vi "GetFilesPCI.vi"(4 "error in (no error)":errorcluster, 6 "Test Num :":u32, 7 "Project :":string) -> (0 "error out":errorcluster, 3 "NomProjetOut":string)   [LabVIEW 2017]
uses:
  DefDeType/WhichPath.ctl
panel:
  out "Glissière":i32(slide) scale=0.0..100.0
  out "noms des fichiers":string[](array[string])
  out "HBM File":bool
  out "Qualisys file":bool
  out "PCI file":bool
  in  "Etat":string
  # "Files Check"
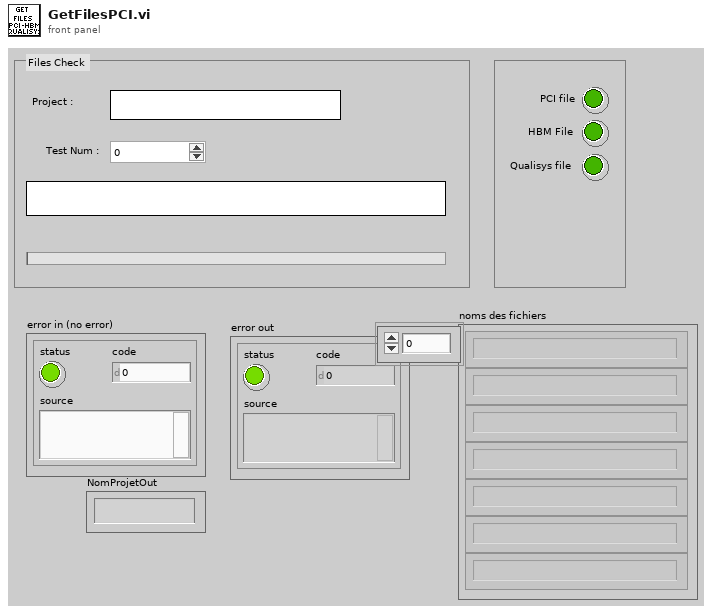
[diagram p1: front panel]
types:
  T1 = typedef "WhichPath.ctl" = enum16{"DossierProjet", "Config", "Meas", "MeasPCI", "MeasCRIO1", "MeasCRIO2", "MeasQualisys", "MeasHBM", "MeasTDMS", "Fig", "Res"}
  T2 = typedef "ConfigTotale.ctl" = cluster{"VoltageChannels":T3, "WheastoneBridgeChannels":T4, "Configuration":T5}
  T3 = typedef "VoltageChannels.ctl" = cluster{"ChannelNames":string[], "Sensitivity(Unit/V)":dbl[], "AutoZero":bool[], "ChannelUnits":string[], "Offsets(Units)":dbl[], "Graph Num":u8[]}
  T4 = typedef "WBridgeChannels.ctl" = cluster{"ChannelNames":string[], "Sensitivity(Unit/V)":dbl[], "AutoZero":bool[], "ChannelUnits":string[], "Offsets(Units)":dbl[], "Graph Num":u8[]}
  T5 = typedef "Configuration.ctl" = cluster{"AcqSamplingRate(Hz)":u32, "AcqTime(s)":u32, "Trigger":bool, "NbVoltageChannels":u32, "NbWBridgeChannels":u32, "Qualisys":bool, "Hexapode":bool, "FinalSamplingRate(Hz)":u32, "QualisysDataType":enum16{"6DOF", "3DTracking", "6DOF + 3D"}, "Nortek":bool, "HBM":bool}
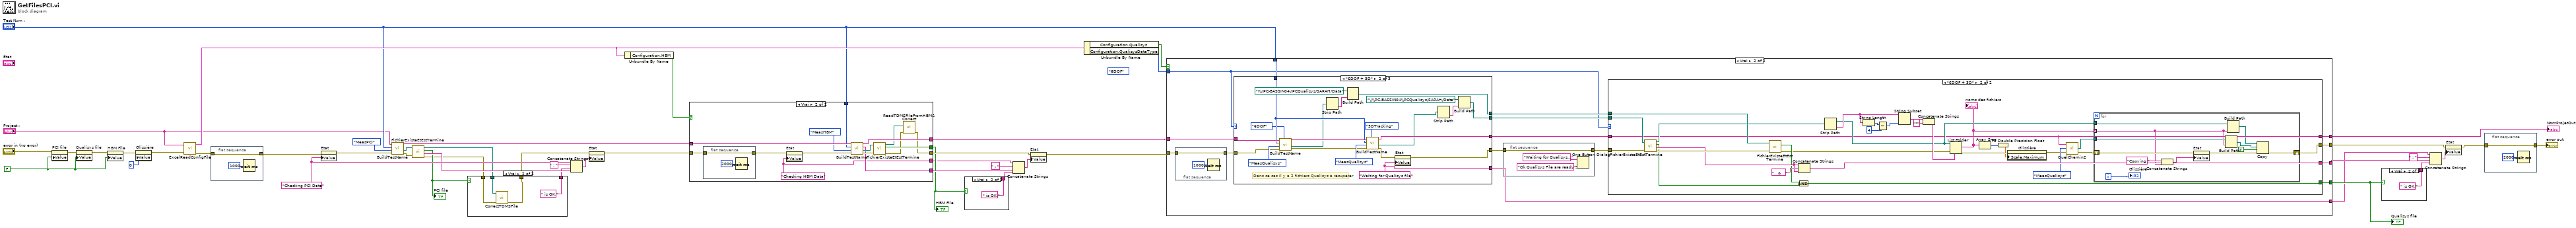
[diagram p0: block diagram]
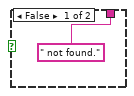
[diagram p2: hidden frame]
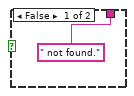
[diagram p3: hidden frame]
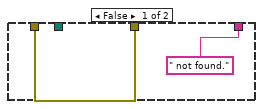
[diagram p4: hidden frame]
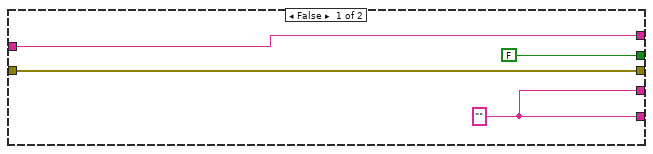
[diagram p5: hidden frame]
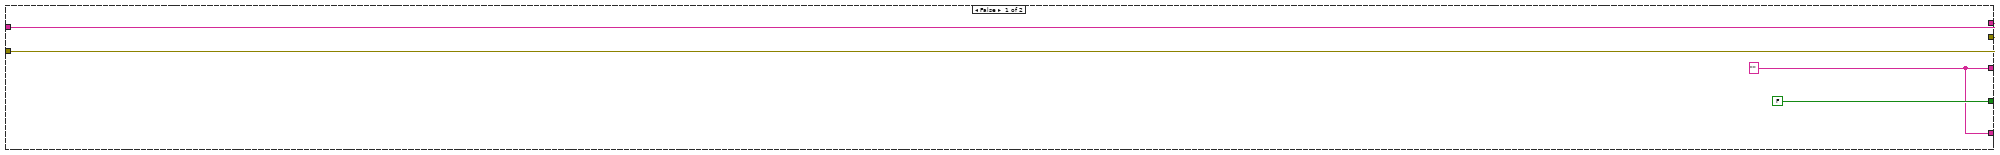
[diagram p6: hidden frame]
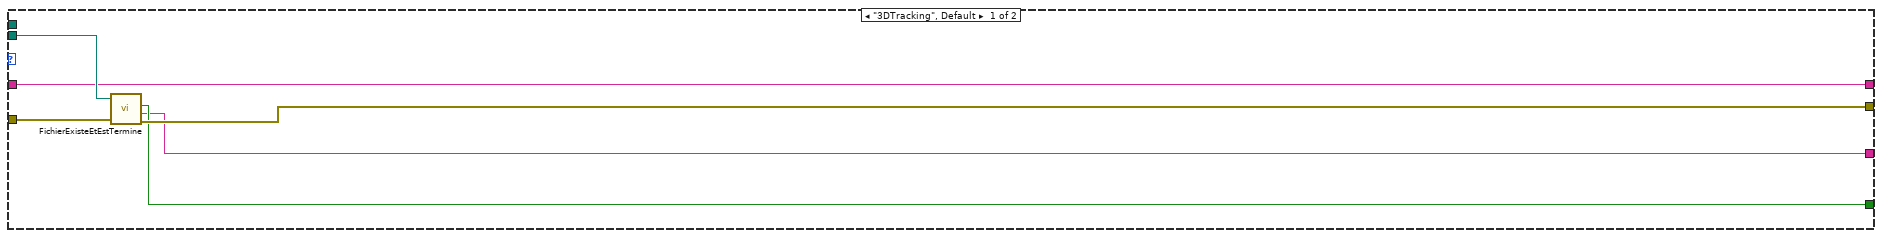
[diagram p7: hidden frame]
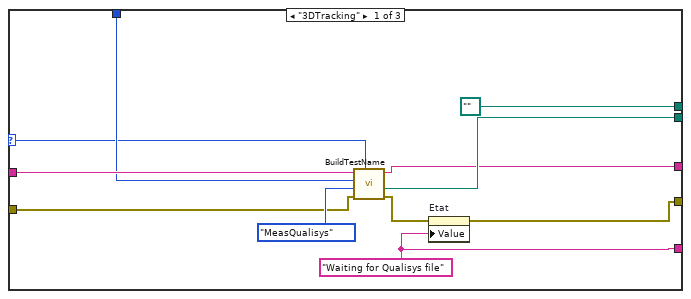
[diagram p8: hidden frame]
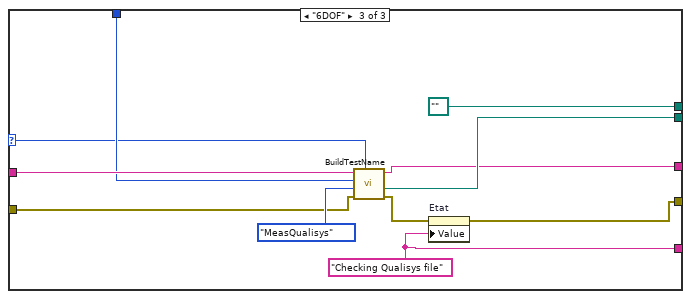
[diagram p9: hidden frame]
diagram:
  w27 = "Checking PCI Data" ("Etat")
  (unwired) enum16{"6DOF", "3DTracking", "6DOF + 3D"}."6DOF" ("Configuration.QualisysDataType")
  w38 = FALSE ("Valise file")
  n1 = property on="PCI file" class="Bool (strict)"(error in="error in (no error)", "Value"=w38) -> (error out=w48:errorcluster)  [unwired: 1 in, 1 out]
  n2 = property on="Qualisys file" class="Bool (strict)"(error in=w48, "Value"=w38) -> (error out=w39:errorcluster)  [unwired: 1 in, 1 out]
  n3 = property on="HBM File" class="Bool (strict)"(error in=w39, "Value"=w38) -> (error out=w3:errorcluster)  [unwired: 1 in, 1 out]
  n4 = property on="Glissière" class="Gliss (strict)"(error in=w3, "Value"=0 ("Glissière")) -> (error out=w2:errorcluster)  [unwired: 1 in, 1 out]
  n5 = call "ExcelReadConfigFile.vi"("NomProjet"="Project :", "error in (no error)"=w2) -> ("ConfigurationTotale"=w41:T2, "error out"=w44:errorcluster)  [unwired: 3 in]
  n6 = flat-sequence {
    tunnel: w44 -> [w51]
    tunnel: [w51] -> w31
    frame #0 {
      n7 = Wait (ms)(milliseconds to wait=u32 1000) -> ()  [unwired: 1 out]
    }
  }
  n8 = property on="Etat" class="Ch"(error in=w31, "Value"=w27) -> (error out=w30:errorcluster)  [unwired: 1 in, 1 out]
  n9 = call "BuildTestName.vi"("entrée d'erreur"=w30, "WhichPath?"=WhichPath."MeasPCI", "NextTestNum"="Test Num :", "NomProjet"="Project :") -> ("sortie d'erreur"=w33:errorcluster, "cheminProchainFichier"=w32:path, "NomProjetOut"=w34:string)  [unwired: 1 in, 1 out]
  n10 = call "FichierExisteEtEstTermine.vi"("cheminProchainFichierRAW"=w32, "entrée d'erreur (pas d'erreur)"=w33) -> ("path out"=w6:path, "ExisteEtTermine"=w23:bool, "nomFichier"=w25:string, "sortie d'erreur"=w5:errorcluster)  [unwired: 1 in]
  "PCI file" <- w23
  n11 = case shown="Vrai" w23 {
    tunnel: [" not found." ("chaîne") " is OK." ("chaîne")] -> w24
    tunnel: w6 -> [_ w54]
    tunnel: w5 -> [w52 w56]
    tunnel: [w52 w55] -> w4
    frame False {
    }
    frame True {
      n12 = call "CorrectTDMSFile.vi"("entrée d'erreur (pas d'erreur)"=w56, "chemin du fichier"=w54) -> ("sortie d'erreur"=w55:errorcluster)  [unwired: 5 in]
    }
  }
  n13 = Concatenate Strings(w27, " : " ("chaîne"), w25, w24) -> (w28:string)
  n14 = property on="Etat" class="Ch"(error in=w4, "Value"=w28) -> (error out=w29:errorcluster)  [unwired: 1 in, 1 out]
  n15 = Unbundle By Name(w41) -> ("Configuration.HBM"=w43:bool)
  n16 = case shown="Vrai" w43 {
    tunnel: w29 -> [w61 w72]
    tunnel: [w61 w63] -> w19
    tunnel: [w60 w70] -> w40
    tunnel: w34 -> [w60 w76]
    tunnel: "Test Num :" -> [_ w74]
    tunnel: [FALSE ("ExisteEtTermine") w67] -> w16
    tunnel: [w58 w66] -> w17
    tunnel: [w58 w65] -> w8
    frame False {
      w58 = "" ("NomProchainFichier")
    }
    frame True {
      w65 = "Checking HBM Data" ("Etat")
      n17 = flat-sequence {
        tunnel: w72 -> [w78]
        tunnel: [w78] -> w73
        frame #0 {
          n18 = Wait (ms)(milliseconds to wait=u32 2000) -> ()  [unwired: 1 out]
        }
      }
      n19 = property on="Etat" class="Ch"(error in=w73, "Value"=w65) -> (error out=w75:errorcluster)  [unwired: 1 in, 1 out]
      n20 = call "BuildTestName.vi"("entrée d'erreur"=w75, "WhichPath?"=WhichPath."MeasHBM", "NextTestNum"=w74, "NomProjet"=w76) -> ("sortie d'erreur"=w68:errorcluster, "cheminProchainFichier"=w69:path, "NomProchainFichier"=w66:string, "NomProjetOut"=w70:string)  [unwired: 1 in]
      n21 = call "FichierExisteEtEstTermine.vi"("cheminProchainFichierRAW"=w69, "entrée d'erreur (pas d'erreur)"=w68) -> ("path out"=w62:path, "ExisteEtTermine"=w67:bool, "sortie d'erreur"=w64:errorcluster)  [unwired: 1 in, 1 out]
      n22 = call "ReadTDMSFileFromHBM&Correct.vi"("error in (no error)"=w64, "file path"=w62) -> ("sortie d'erreur"=w63:errorcluster)  [unwired: 4 in, 1 out]
    }
  }
  "HBM File" <- w16
  n23 = case shown="Vrai" w16 {
    tunnel: [" not found." ("chaîne") " is OK." ("chaîne")] -> w22
    frame False {
    }
    frame True {
    }
  }
  n24 = Concatenate Strings(w8, " : " ("chaîne"), w17, w22) -> (w20:string)
  n25 = property on="Etat" class="Ch"(error in=w19, "Value"=w20) -> (error out=w18:errorcluster)  [unwired: 1 in, 1 out]
  n26 = Unbundle By Name(w41) -> ("Configuration.Qualisys"=w47:bool, "Configuration.QualisysDataType"=w45:enum16{"6DOF", "3DTracking", "6DOF + 3D"})
  n27 = case shown="Vrai" w47 {
    tunnel: w18 -> [w84 w93]
    tunnel: w40 -> [w83 w97]
    tunnel: w45 -> [_ w90]
    tunnel: "Test Num :" -> [_ w96]
    tunnel: [w84 w95] -> w12
    tunnel: [w83 w94] -> w42
    tunnel: [w81 w87] -> w10
    tunnel: [FALSE ("ExisteEtTermine") w89] -> w9
    tunnel: [w81 w88] -> w7
    frame False {
      w81 = "" ("nomFichier")
    }
    frame True {
      n28 = flat-sequence {
        tunnel: w93 -> [w195]
        tunnel: [w195] -> w92
        frame #0 {
          n29 = Wait (ms)(milliseconds to wait=u32 1000) -> ()  [unwired: 1 out]
        }
      }
      n30 = case shown="\"6DOF + 3D\"" w90 {
        selector: w90 -> [w153 _ w185]
        tunnel: [w161 w162 w193] -> w99
        tunnel: [w160 w182 w192] -> w86
        tunnel: [w159 w181 w191] -> w98
        tunnel: w97 -> [w156 w174 w188]
        tunnel: w96 -> [w155 w173 w187]
        tunnel: w92 -> [w154 w176 w186]
        tunnel: [path "" ("cheminProchainFichier") w166 path "" ("cheminProchainFichier")] -> w91
        tunnel: [w151 w170 w183] -> w88
        frame "3DTracking" {
          w151 = "Waiting for Qualisys file" ("Etat")
          n31 = call "BuildTestName.vi"("QualisysDataType"=w153, "entrée d'erreur"=w154, "WhichPath?"=WhichPath."MeasQualisys", "NextTestNum"=w155, "NomProjet"=w156) -> ("sortie d'erreur"=w157:errorcluster, "cheminProchainFichier"=w161:path, "NomProjetOut"=w159:string)  [unwired: 1 out]
          n32 = property on="Etat" class="Ch"(error in=w157, "Value"=w151) -> (error out=w160:errorcluster)  [unwired: 1 in, 1 out]
        }
        frame "6DOF + 3D" {
          w170 = "Waiting for Qualisys file" ("Etat")
          # "Dans ce cas il y a 2 fichiers Qualisys à récupérer"
          n33 = call "BuildTestName.vi"("QualisysDataType"=enum16{"6DOF", "3DTracking", "6DOF + 3D"}."6DOF", "entrée d'erreur"=w176, "WhichPath?"=WhichPath."MeasQualisys", "NextTestNum"=w173, "NomProjet"=w174) -> ("sortie d'erreur"=w177:errorcluster, "cheminProchainFichier"=w168:path, "NomProjetOut"=w175:string)  [unwired: 1 out]
          n34 = Strip Path(path=w168) -> (name=w167:string)  [unwired: 1 out]
          n35 = Build Path(base path=path "\\\\PC-BASSIN04\\PCQualisys/SARAH/Data" ("chemin de base"), name or relative path=w167) -> (appended path=w166:path)
          n36 = call "BuildTestName.vi"("QualisysDataType"=enum16{"6DOF", "3DTracking", "6DOF + 3D"}."3DTracking", "entrée d'erreur"=w177, "WhichPath?"=WhichPath."MeasQualisys", "NextTestNum"=w173, "NomProjet"=w175) -> ("sortie d'erreur"=w179:errorcluster, "cheminProchainFichier"=w163:path, "NomProjetOut"=w181:string)  [unwired: 1 out]
          n37 = property on="Etat" class="Ch"(error in=w179, "Value"=w170) -> (error out=w182:errorcluster)  [unwired: 1 in, 1 out]
          n38 = Strip Path(path=w163) -> (name=w165:string)  [unwired: 1 out]
          n39 = Build Path(base path=path "\\\\PC-BASSIN04\\PCQualisys/SARAH/Data" ("chemin de base"), name or relative path=w165) -> (appended path=w162:path)
        }
        frame "6DOF" {
          w183 = "Checking Qualisys file" ("Etat")
          n40 = call "BuildTestName.vi"("QualisysDataType"=w185, "entrée d'erreur"=w186, "WhichPath?"=WhichPath."MeasQualisys", "NextTestNum"=w187, "NomProjet"=w188) -> ("sortie d'erreur"=w189:errorcluster, "cheminProchainFichier"=w193:path, "NomProjetOut"=w191:string)  [unwired: 1 out]
          n41 = property on="Etat" class="Ch"(error in=w189, "Value"=w183) -> (error out=w192:errorcluster)  [unwired: 1 in, 1 out]
        }
      }
      n42 = flat-sequence {
        tunnel: w86 -> [w102]
        tunnel: [w102] -> w85
        frame #0 {
          n43 = One Button Dialog(message="Waiting for Qualisys...", button name ("OK")="Ok Qualisys File are ready!!" ("nom du bouton (\"OK\")")) -> ()  [unwired: 1 out]
        }
      }
      n44 = case shown="\"6DOF + 3D\"" w90 {
        tunnel: w99 -> [w107 w136]
        tunnel: w85 -> [w108 w138]
        tunnel: w98 -> [w105 w117]
        tunnel: [w106 w120] -> w95
        tunnel: [w105 w117] -> w94
        tunnel: w91 -> [_ w135]
        tunnel: [w104 w129] -> w89
        tunnel: [w103 w132] -> w87
        frame "3DTracking", Default {
          n45 = call "FichierExisteEtEstTermine.vi"("cheminProchainFichierRAW"=w107, "entrée d'erreur (pas d'erreur)"=w108) -> ("ExisteEtTermine"=w104:bool, "nomFichier"=w103:string, "sortie d'erreur"=w106:errorcluster)  [unwired: 1 in, 1 out]
        }
        frame "6DOF + 3D" {
          n46 = call "FichierExisteEtEstTermine.vi"("cheminProchainFichierRAW"=w136, "entrée d'erreur (pas d'erreur)"=w138) -> ("path out"=w128:path, "ExisteEtTermine"=w130:bool, "nomFichier"=w133:string, "sortie d'erreur"=w137:errorcluster)  [unwired: 1 in]
          n47 = call "FichierExisteEtEstTermine.vi"("cheminProchainFichierRAW"=w135, "entrée d'erreur (pas d'erreur)"=w137) -> ("ExisteEtTermine"=w131:bool, "sortie d'erreur"=w112:errorcluster)  [unwired: 1 in, 2 out]
          n48 = And(x=w131, y=w130) -> (x .and. y?=w129:bool)
          n49 = Concatenate Strings(w133, "   &   " ("chaîne"), w133) -> (w132:string)
          n50 = Strip Path(path=w128) -> (stripped path=w119:path, name=w127:string)
          n51 = String Length(string=w127) -> (length=w126:i32)
          n52 = Subtract(x=w126, y=4) -> (x-y=w124:i32)
          n53 = String Subset(string=w127, length (rest)=w124) -> (substring=w123:string)  [unwired: 1 in]
          n54 = Concatenate Strings(w123, "*" ("chaîne")) -> (w121:string)
          n55 = List Folder(path=w119, pattern=w121, error in=w112) -> (filenames=w111:string[], error out=w113:errorcluster)  [unwired: 1 in, 2 out]
          "noms des fichiers" <- w111
          n56 = Array Size(array=w111) -> (size(s)=w110:i32)
          n57 = To Double Precision Float(number=w110) -> (double precision float=w109:dbl)
          n58 = property on="Glissière" class="Gliss (strict)"(error in=w113, "Scale.Maximum"=w109) -> (error out=w114:errorcluster)  [unwired: 1 in, 1 out]
          n59 = call "QuelChemin2.vi"("Entrée d'erreur"=w114, "WhichPath?"=WhichPath."MeasQualisys", "NomProjet"=w117) -> ("Sortie d'erreur"=w118:errorcluster, "SurDisqueReseau"=w115:path)  [unwired: 1 out]
          n60 = for {
            tunnel: w111 -> [w141] mode=indexing
            shift-right: [w149] -> w120
            shift-left: w118 -> [w144]
            tunnel: w119 -> [w150]
            tunnel: w115 -> [w146]
            i -> [w139]
            n61 = Concatenate Strings("Copying " ("Etat"), w141) -> (w140:string)
            n62 = property on="Etat" class="Ch"(error in=w144, "Value"=w140) -> (error out=w143:errorcluster)  [unwired: 1 in, 1 out]
            n63 = Build Path(base path=w146, name or relative path=w141) -> (appended path=w145:path)
            n64 = Build Path(base path=w150, name or relative path=w141) -> (appended path=w148:path)
            n65 = Copy(8:w143, 9:TRUE ("écraser (F)"), 10:w145, 11:w148) -> (0:w149:errorcluster)  [unwired: 1 in, 2 out]
            "Glissière" <- w139
          }
        }
      }
    }
  }
  "Qualisys file" <- w9
  "NomProjetOut" <- w42
  n66 = case shown="Vrai" w9 {
    tunnel: [" not found." ("chaîne") " is OK." ("chaîne")] -> w13
    frame False {
    }
    frame True {
    }
  }
  n67 = Concatenate Strings(w7, " : " ("chaîne"), w10, w13) -> (w15:string)
  n68 = property on="Etat" class="Ch"(error in=w12, "Value"=w15) -> (error out=w11:errorcluster)  [unwired: 1 in, 1 out]
  n69 = flat-sequence {
    tunnel: w11 -> [w199]
    tunnel: [w199] -> w46
    frame #0 {
      n70 = Wait (ms)(milliseconds to wait=u32 2000) -> ()  [unwired: 1 out]
    }
  }
  "error out" <- w46
